vi "ESN_outputCompare.vi"(8 "Time settings":cluster{"t start":i32, "t length":i32}={"t start"=0, "t length"=2147483647}, 9 "index (row)":i32, 10 "disired output":dbl[][](array[numeric]), 11 "output":dbl[][](array[numeric])) -> (3 "Waveform Graph":dbl[][](graph))   [LabVIEW 2017]
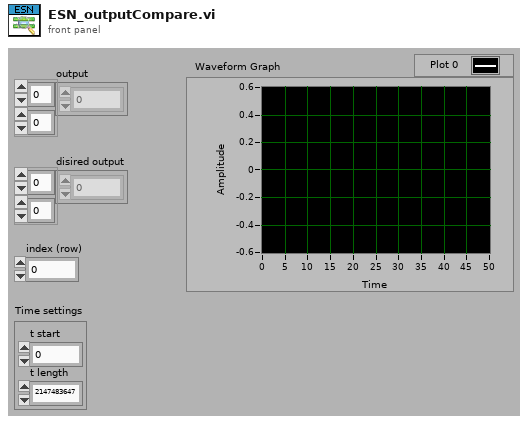
[diagram p1: front panel]
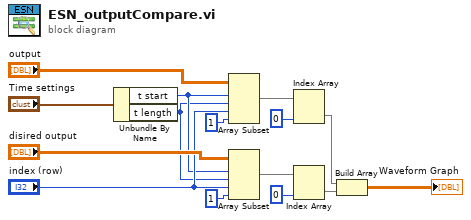
[diagram p0: block diagram]
diagram:
  n1 = Unbundle By Name("Time settings") -> ("t start"=w5:i32, "t length"=w4:i32)
  n2 = Array Subset(array="output", index (row)=w5, length (row)=w4, index (col)="index (row)", length (col)=1 ("length")) -> (w3:dbl[][])
  n3 = Array Subset(array="disired output", index (row)=w5, length (row)=w4, index (col)="index (row)", length (col)=1 ("length")) -> (w12:dbl[][])
  n4 = Index Array(array=w3, index (col)=0 ("disabled index (col)")) -> (element=w13:dbl[])  [unwired: 1 in]
  n5 = Index Array(array=w12, index (col)=0 ("disabled index (col)")) -> (element=w10:dbl[])  [unwired: 1 in]
  n6 = Build Array(w13, w10) -> (→"Waveform Graph":dbl[][])
